vi "Write Connections.vi"(8 "error in (no error)":errorcluster, 10 "Connections":T1={"GEN-SYS VISA resource name"="", "OVG-4"={"Flow Address"=2, "Temp Address"=1}, "OHG-4"={"Flow Address"=2, "Easydew VISA resource name"=""}}, 11 "Owlstone OVG-4 in":refnum<class "Owlstone GEN-SYS.lvclass">) -> (0 "error out":errorcluster, 3 "Owlstone OVG-4 out":refnum<class "Owlstone GEN-SYS.lvclass">)   [LabVIEW 2011, in "Owlstone GEN-SYS.lvclass"]
uses:
  Owlstone GEN-SYS.lvclass
  GEN-SYS Connections.ctl
  Owlstone GEN-SYS.lvclass/Owlstone GEN-SYS.ctl
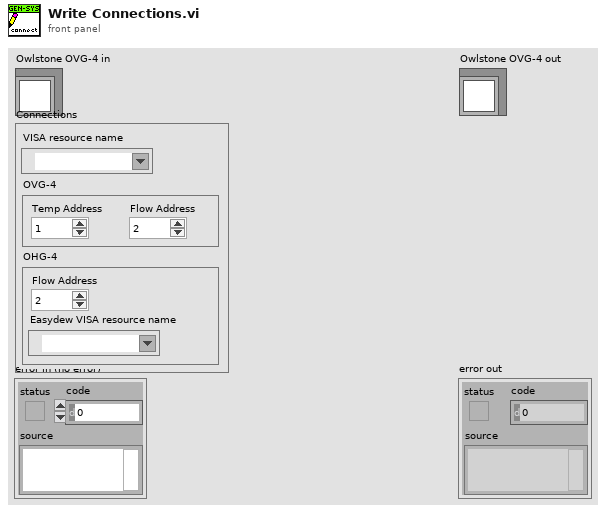
[diagram p1: front panel]
types:
  T1 = typedef "Owlstone GEN-SYS.lvclass/GEN-SYS Connections.ctl" = cluster{"GEN-SYS VISA resource name":refnum<visa-resource-name>, "OVG-4":cluster{"Flow Address":u8, "Temp Address":u8}, "OHG-4":cluster{"Flow Address":u8, "Easydew VISA resource name":refnum<visa-resource-name>}}
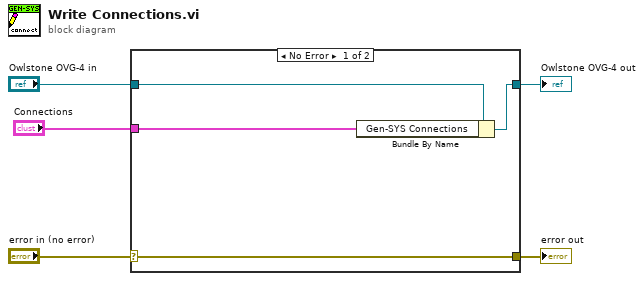
[diagram p0: block diagram]
diagram:
  n1 = case shown="No Error" "error in (no error)" {
    selector: "error in (no error)" -> [w9 w10]
    tunnel: [w9 w10] -> w4
    tunnel: [w7 w11] -> w2
    tunnel: "Owlstone OVG-4 in" -> [w8 w11]
    tunnel: "Connections" -> [w6 _]
    frame No Error {
      n2 = Bundle By Name(cluster=w8, "Gen-SYS Connections"=w6) -> (w7:refnum<class "Owlstone GEN-SYS.lvclass">)
    }
    frame Error {
    }
  }
  "error out" <- w4
  "Owlstone OVG-4 out" <- w2
